vi "PLC_comm.vi"() -> ()   [LabVIEW 2017]
uses:
  <vilib>/DATA AHEAD/SP7/typedefs/PLC Type.ctl
  <vilib>/Utility/error.llb/DialogType.ctl
  <vilib>/addons/database/Connection.llb/DB Tools Open Connec (String).vi
  Global/Global 1.vi
  Global/DATA LOG.vi
  <vilib>/DATA AHEAD/SP7/functions/write/write Dint array.vi
  <vilib>/DATA AHEAD/SP7/functions/write/writeString.vi
  <vilib>/DATA AHEAD/SP7/functions/read/read Dint array.vi
  <vilib>/DATA AHEAD/SP7/functions/read/read real array.vi
  <vilib>/DATA AHEAD/SP7/functions/read/read String.vi
  <vilib>/addons/database/NI_Database_API.lvlib
  <vilib>/DATA AHEAD/SP7/SP7.lvlib
panel:
  out "IP1 7":string
  out "PLC 7":bool
  out "IP1 6":string
  out "PLC 6":bool
  out "IP1 5":string
  out "PLC 5":bool
  out "PLC 4":bool
  out "PLC 3":bool
  out "PLC 2":bool
  out "PLC 1":bool
  out "IP1 4":string
  out "IP1 3":string
  out "IP1 2":string
  out "IP1":string
  in  "stop":bool
  out "error out":errorcluster
  in  "error in (no error)":errorcluster
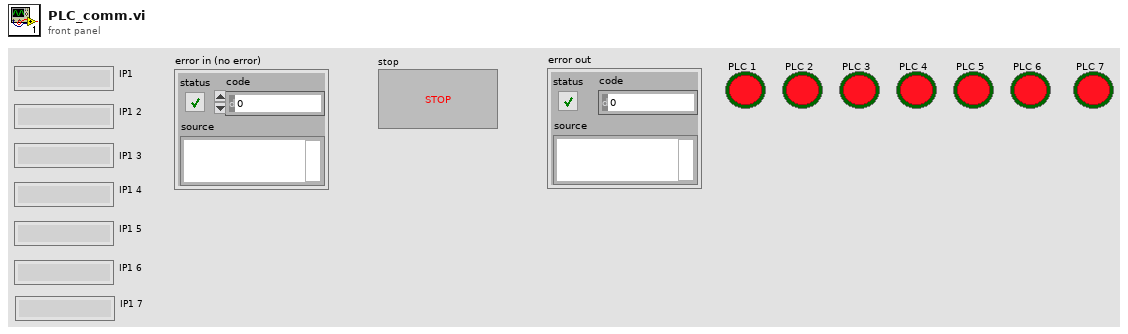
[diagram p1: front panel]
types:
  T1 = typedef "DialogType.ctl" = u16
  T2 = typedef "SP7.lvlib/PLC Type.ctl" = enum16{"S7 200", "S7 300/400", "S7 1200", "S7 1500", "LOGO!8"}
  T3 = typedef "NI_Database_API.lvlib/Conn ObjectReference.ctl" = refnum<k1>
  T4 = typedef "SP7.lvlib/S7 Connection.ctl" = cluster{"TCP Connection Ref":refnum<k5>, "IP address":string, "timeout ms":i32, "Connected?":bool, "PLC Type":T2, "Rack S7 400":u8, "Slot S7 400":u8, "PDU Size":u16, "connection semaphore":T5}
  T5 = typedef "Semaphore RefNum" = refnum<k1>
diagram:
  w2 = T1 0 items=["no dialog", "OK message", "continue or stop message", "OK message + warnings", "continue/stop + warnings"]  # type of dialog (OK msg:1)
  w4 = i32[] [0, 0, 0, 0, 0]  # I/P
  w5 = i32[] [0, 0]  # Input
  w7 = i32[] [0, 0]  # Input
  w8 = i32[] [0, 0]  # Input
  w10 = i32[] [0, 0]  # Input
  w6 = i32[] [0, 0, 0, 0, 0]  # I/P
  w9 = i32[] [0, 0, 0, 0, 0]  # I/P
  w11 = i32[] [0, 0, 0, 0, 0]  # I/P
  w12 = i32[] [0, 0, 0, 0, 0]  # I/P
  w13 = i32[] [0, 0]  # Input
  w14 = i32[] [0, 0]  # Input
  w15 = i32[] [0, 0, 0, 0, 0]  # I/P
  w16 = i32[] [0, 0, 0, 0, 0]  # I/P
  w17 = i32[] [0, 0]  # Input
  w18 = i32[] [0, 0]  # I/P
  w19 = i32[] [0, 0]  # Input
  # "OP 80"
  # "OP 70"
  # "OP 60"
  # "OP 50"
  # "OP 40"
  # "OP 30"
  # "OP 20"
  # "OP 10"
  n1 = call "path_db.vi"("error in"="error in (no error)") -> ("error out"=w174:errorcluster, "resulting string"=w179:string)  [unwired: 9 in]
  n2 = call-poly <vilib>:"DB Tools Open Connection.vi"("error in (no error)"=w174, "connection information"=w179) -> ("error out"=w178:errorcluster, "connection reference"=w177:T3)  [unwired: 6 in]
  n3 = call <vilib>:"DB Tools Select Data.vi"("error in (no error)"=w178, "columns"=string[] ["PLC_IP_1", "PLC_IP_2", "PLC_IP_3", "PLC_IP_4", "PLC_IP_5", "PLC_IP_6", "PLC_IP_7"], "table"="IP_SETTING", "connection reference"=w177) -> ("error out"=w176:errorcluster, "data"=w175:variant[][])  [unwired: 2 in, 1 out]
  n4 = call "PADMINI_varient_to_data.vi"("error in (no error)"=w176, "data"=w175) -> ("error out"=w26:errorcluster, "Array"=w170:string[][])  [unwired: 8 in]
  n5 = call "PADMINI_AUTO_CYCLE STATE.vi"("Enum"=enum16{"Read", "Write"}."Write", "error in (no error)"=w26, "Input"=w19) -> ("error out"=w156:errorcluster)  [unwired: 7 in, 1 out]
  n6 = Index Array(array=w170, index (row)=0) -> (element=w169:string[])  [unwired: 1 in]
  n7 = call "PADMINI_AUTO_BARCODE_STRING.vi"("Enum"=enum16{"Read", "Write"}."Write", "error in (no error)"=w156, "Input"=string[] ["", ""]) -> ("error out"=w153:errorcluster)  [unwired: 7 in, 1 out]
  n8 = call "PADMINI_AUTO_BARCODE_STATUS.vi"("Enum"=enum16{"Read", "Write"}."Write", "error in (no error)"=w153, "I/P"=w18) -> ("error out"=w151:errorcluster)  [unwired: 7 in, 1 out]
  n9 = call "PADMINI_AUTO_CYCLE VALUE 10.vi"("Enum"=enum16{"Read", "Write"}."Write", "error in (no error)"=w151, "Input"=dbl[] [0.0]) -> ("error out"=w145:errorcluster)  [unwired: 7 in, 1 out]
  n10 = call "PADMINI_AUTO_CYCLE STATE 20.vi"("Enum"=enum16{"Read", "Write"}."Write", "error in (no error)"=w145, "Input"=w5) -> ("error out"=w143:errorcluster)  [unwired: 7 in, 1 out]
  n11 = call "PADMINI_AUTO_CYCLE VALUE 20.vi"("Enum"=enum16{"Read", "Write"}."Write", "error in (no error)"=w143, "Input"=dbl[] [0.0, 0.0, 0.0, 0.0]) -> ("error out"=w139:errorcluster)  [unwired: 7 in, 1 out]
  n12 = call "PADMINI_AUTO_BARCODE_STRING2.vi"("Enum"=enum16{"Read", "Write"}."Write", "error in (no error)"=w139, "Input"=string[] ["", "", "", "", "", "", ""]) -> ("error out"=w137:errorcluster)  [unwired: 7 in, 1 out]
  n13 = call "PADMINI_AUTO_BARCODE_STATUS 20.vi"("Enum"=enum16{"Read", "Write"}."Write", "error in (no error)"=w137, "I/P"=w4) -> ("error out"=w131:errorcluster)  [unwired: 7 in, 1 out]
  n14 = call "PADMINI_AUTO_BARCODE_STATUS 30.vi"("Enum"=enum16{"Read", "Write"}."Write", "error in (no error)"=w131, "I/P"=w6) -> ("error out"=w128:errorcluster)  [unwired: 7 in, 1 out]
  n15 = call "PADMINI_AUTO_CYCLE STATE 30.vi"("Enum"=enum16{"Read", "Write"}."Write", "error in (no error)"=w128, "Input"=w7) -> ("error out"=w127:errorcluster)  [unwired: 7 in, 1 out]
  n16 = call "PADMINI_AUTO_CYCLE VALUE 30.vi"("Enum"=enum16{"Read", "Write"}."Write", "error in (no error)"=w127, "Input"=dbl[] [0.0, 0.0]) -> ("error out"=w124:errorcluster)  [unwired: 7 in, 1 out]
  n17 = call "PADMINI_AUTO_BARCODE_STRING 30.vi"("Enum"=enum16{"Read", "Write"}."Write", "error in (no error)"=w124, "Input"=string[] ["", "", ""]) -> ("error out"=w102:errorcluster)  [unwired: 7 in, 1 out]
  n18 = call "PADMINI_AUTO_BARCODE_STATUS 40.vi"("Enum"=enum16{"Read", "Write"}."Write", "error in (no error)"=w102, "I/P"=w9) -> ("error out"=w101:errorcluster)  [unwired: 7 in, 1 out]
  n19 = call "PADMINI_AUTO_CYCLE VALUE 40.vi"("Enum"=enum16{"Read", "Write"}."Write", "error in (no error)"=w101, "Input"=dbl[] [0.0, 0.0, 0.0, 0.0]) -> ("error out"=w100:errorcluster)  [unwired: 7 in, 1 out]
  n20 = call "PADMINI_AUTO_CYCLE STATE 40.vi"("Enum"=enum16{"Read", "Write"}."Write", "error in (no error)"=w100, "Input"=w8) -> ("error out"=w99:errorcluster)  [unwired: 7 in, 1 out]
  n21 = call "PADMINI_AUTO_BARCODE_STRING 40.vi"("Enum"=enum16{"Read", "Write"}."Write", "error in (no error)"=w99, "Input"=string[] ["", "", "", "", ""]) -> ("error out"=w81:errorcluster)  [unwired: 7 in, 1 out]
  n22 = call "PADMINI_AUTO_BARCODE_STATUS 50.vi"("Enum"=enum16{"Read", "Write"}."Write", "error in (no error)"=w81, "I/P"=w11) -> ("error out"=w83:errorcluster)  [unwired: 7 in, 1 out]
  n23 = call "PADMINI_AUTO_CYCLE STATE 50.vi"("Enum"=enum16{"Read", "Write"}."Write", "error in (no error)"=w83, "Input"=w10) -> ("error out"=w87:errorcluster)  [unwired: 7 in, 1 out]
  n24 = call "PADMINI_AUTO_CYCLE VALUE 50.vi"("Enum"=enum16{"Read", "Write"}."Write", "error in (no error)"=w87, "Input"=dbl[] [0.0, 0.0, 0.0]) -> ("error out"=w84:errorcluster)  [unwired: 7 in, 1 out]
  n25 = call "PADMINI_AUTO_BARCODE_STRING 50.vi"("Enum"=enum16{"Read", "Write"}."Write", "error in (no error)"=w84, "Input"=string[] ["", "", "", ""]) -> ("error out"=w59:errorcluster)  [unwired: 7 in, 1 out]
  n26 = call "PADMINI_AUTO_BARCODE_STATUS 60.vi"("Enum"=enum16{"Read", "Write"}."Write", "error in (no error)"=w59, "I/P"=w12) -> ("error out"=w63:errorcluster)  [unwired: 7 in, 1 out]
  n27 = call "PADMINI_AUTO_CYCLE STATE 60.vi"("Enum"=enum16{"Read", "Write"}."Write", "error in (no error)"=w63, "Input"=w13) -> ("error out"=w65:errorcluster)  [unwired: 7 in, 1 out]
  n28 = call "PADMINI_AUTO_CYCLE VALUE 60.vi"("Enum"=enum16{"Read", "Write"}."Write", "error in (no error)"=w65, "Input"=dbl[] [0.0, 0.0, 0.0, 0.0, 0.0]) -> ("error out"=w68:errorcluster)  [unwired: 7 in, 1 out]
  n29 = call "PADMINI_AUTO_BARCODE_STRING 60.vi"("Enum"=enum16{"Read", "Write"}."Write", "error in (no error)"=w68, "Input"=string[] ["", "", "", "", "", ""]) -> ("error out"=w35:errorcluster)  [unwired: 7 in, 1 out]
  n30 = call "PADMINI_AUTO_BARCODE_STATUS 70.vi"("Enum"=enum16{"Read", "Write"}."Write", "error in (no error)"=w35, "I/P"=w15) -> ("error out"=w38:errorcluster)  [unwired: 7 in, 1 out]
  n31 = call "PADMINI_AUTO_CYCLE STATE 70.vi"("Enum"=enum16{"Read", "Write"}."Read", "error in (no error)"=w38, "Input"=w14) -> ("error out"=w50:errorcluster)  [unwired: 7 in, 1 out]
  n32 = call "PADMINI_AUTO_CYCLE VALUE 70.vi"("Enum"=enum16{"Read", "Write"}."Write", "error in (no error)"=w50, "Input"=dbl[] [0.0, 0.0]) -> ("error out"=w47:errorcluster)  [unwired: 7 in, 1 out]
  n33 = call "PADMINI_AUTO_BARCODE_STRING 70.vi"("Enum"=enum16{"Read", "Write"}."Write", "error in (no error)"=w47, "Input"=string[] ["", ""]) -> ("error out"=w32:errorcluster)  [unwired: 7 in, 1 out]
  n34 = call "PADMINI_AUTO_BARCODE_STATUS 80.vi"("Enum"=enum16{"Read", "Write"}."Write", "error in (no error)"=w32, "I/P"=w16) -> ("error out"=w39:errorcluster)  [unwired: 7 in, 1 out]
  n35 = call "PADMINI_AUTO_CYCLE STATE 80.vi"("Enum"=enum16{"Read", "Write"}."Write", "error in (no error)"=w39, "Input"=w17) -> ("error out"=w43:errorcluster)  [unwired: 7 in, 1 out]
  n36 = call "PADMINI_AUTO_CYCLE VALUE 80.vi"("Enum"=enum16{"Read", "Write"}."Write", "error in (no error)"=w43, "Input"=sgl[] [0.0]) -> ("error out"=w46:errorcluster)  [unwired: 7 in, 1 out]
  n37 = call "PADMINI_AUTO_BARCODE_STRING 80.vi"("Enum"=enum16{"Read", "Write"}."Write", "error in (no error)"=w46, "Input"=string[] ["", "", ""]) -> ()  [unwired: 7 in, 2 out]
  n38 = Index Array(array=w169) -> (element #1=w118:string, element #2=w119:string, element #3=w113:string, element #4=w89:string, element #5=w71:string, element #6=w28:string, element #7=w27:string)  [unwired: 7 in]
  "IP1" <- w118
  "IP1 2" <- w119
  "IP1 3" <- w113
  "IP1 4" <- w89
  "IP1 5" <- w71
  "IP1 6" <- w28
  "IP1 7" <- w27
  n39 = call <vilib>:"connect.vi"("PLC Type"=PLC_Type."S7 1200" ("PLC Type 2"), "error in (no error)"=w26, "timeout [ms]"=1000 ("timeout [ms] 2"), "IP address"=w27) -> ("error out"=w29:errorcluster, "S7 Connection out"=w1:T4)  [unwired: 6 in]
  n40 = call <vilib>:"connect.vi"("PLC Type"=PLC_Type."S7 1200" ("PLC Type 2"), "error in (no error)"=w26, "timeout [ms]"=1000 ("timeout [ms] 2"), "IP address"=w71) -> ("error out"=w76:errorcluster, "S7 Connection out"=w75:T4)  [unwired: 6 in]
  n41 = call <vilib>:"connect.vi"("PLC Type"=PLC_Type."S7 1200" ("PLC Type 2"), "error in (no error)"=w26, "timeout [ms]"=1000 ("timeout [ms] 2"), "IP address"=w28) -> ("error out"=w56:errorcluster, "S7 Connection out"=w55:T4)  [unwired: 6 in]
  n42 = call <vilib>:"connect.vi"("PLC Type"=PLC_Type."S7 1200" ("PLC Type 2"), "error in (no error)"=w26, "timeout [ms]"=1000 ("timeout [ms] 2"), "IP address"=w89) -> ("error out"=w92:errorcluster, "S7 Connection out"=w93:T4)  [unwired: 6 in]
  n43 = call <vilib>:"connect.vi"("PLC Type"=PLC_Type."S7 1200" ("PLC Type 2"), "error in (no error)"=w26, "timeout [ms]"=1000 ("timeout [ms] 2"), "IP address"=w119) -> ("error out"=w134:errorcluster, "S7 Connection out"=w133:T4)  [unwired: 6 in]
  n44 = call <vilib>:"connect.vi"("PLC Type"=PLC_Type."S7 1200" ("PLC Type 2"), "error in (no error)"=w26, "timeout [ms]"=1000 ("timeout [ms] 2"), "IP address"=w113) -> ("error out"=w115:errorcluster, "S7 Connection out"=w114:T4)  [unwired: 6 in]
  n45 = call <vilib>:"connect.vi"("PLC Type"=PLC_Type."S7 1200" ("PLC Type 2"), "error in (no error)"=w26, "timeout [ms]"=1000, "IP address"=w118) -> ("error out"=w160:errorcluster, "S7 Connection out"=w159:T4)  [unwired: 6 in]
  n46 = while {
    shift-right: [w182] -> w23
    shift-left: w1 -> [w192]
    shift-right: [w190] -> w24
    shift-left: w29 -> [w191]
    tunnel: w27 -> [w181]
    stop <- w184 stop-if-true
    # "OP 90 - 100 - 110"
    n47 = flat-sequence {
      tunnel: [w267] -> w188
      tunnel: [w268] -> w183
      tunnel: w191 -> [w306]
      tunnel: w192 -> [w305]
      tunnel: w181 -> [w287]
      tunnel: [w287] -> w180
      tunnel: [w374] -> w190
      tunnel: [w373] -> w182
      tunnel: w188 -> [w376]
      tunnel: w183 -> [w375]
      tunnel: w180 -> [w372]
      frame #0 {
        w208 = u16 75 ("Data Block #")
        (unwired) u16 1 ("Items # [byte]")
        w233 = u16 72 ("Data Block #")
        w259 = u16 70 ("Data Block #")
        w217 = u16 71 ("Data Block #")
        w247 = u16 69 ("Data Block #")
        # "OP100 OK\nOP 100 NG"
        # "AUTO WRITE"
        n48 = global read "DATA LOG.vi" "OP 90 Outputs"() -> (w304:bool)
        n49 = case shown="True" w304 {
          tunnel: w305 -> [w357 w370]
          tunnel: [w358 w359] -> w264
          tunnel: [w357 w360] -> w265
          tunnel: w306 -> [w358 w367]
          frame False {
          }
          frame True {
            w371 = u16 70  # Data Block #
            n50 = call "PADMINI_AUTO_BARCODE_STATUS 90.vi"("Enum"=enum16{"Read", "Write"}."Read", "error in (no error)"=w367) -> ("error out"=w366:errorcluster, "O/P"=w368:i32[])  [unwired: 8 in]
            n51 = global write "DATA LOG.vi" "OP 90 Outputs"(FALSE) -> ()
            n52 = call-poly <vilib>:"write DB.vi"("DINT input array"=w368, "error in (no error)"=w366, "Data Block #"=w371, "S7 Connection in"=w370) -> ("error out"=w362:errorcluster, "S7 Connection out"=w361:T4)  [unwired: 4 in, 2 out]
            n53 = call-poly <vilib>:"write DB.vi"("DINT input array"=i32[] [0] ("Data Byte"), "error in (no error)"=w362, "Data Block #"=u16 69, "S7 Connection in"=w361) -> ("error out"=w359:errorcluster, "S7 Connection out"=w360:T4)  [unwired: 4 in, 2 out]
          }
        }
        n54 = global read "DATA LOG.vi" "OP 90 reset"() -> (w263:bool)
        n55 = case shown="True" w263 {
          tunnel: w264 -> [w332 w341]
          tunnel: [w332 w340] -> w252
          tunnel: w265 -> [w333 w339]
          tunnel: [w333 w338] -> w253
          frame False {
          }
          frame True {
            n56 = global write "DATA LOG.vi" "OP 90 reset"(FALSE) -> ()
            n57 = call-poly <vilib>:"write DB.vi"("Item offset [byte]"=u16 4 ("Data Block #"), "DINT input array"=i32[] [0], "error in (no error)"=w341, "Data Block #"=u16 69, "S7 Connection in"=w339) -> ("error out"=w340:errorcluster, "S7 Connection out"=w338:T4)  [unwired: 3 in, 2 out]
          }
        }
        n58 = global read "DATA LOG.vi" "Auto Cycle On"() -> (w199:bool)
        n59 = Boolean To (0,1)(Boolean=w199) -> (0, 1=w198:i16)
        n60 = Build Array(w198) -> (w197:i16[])
        n61 = global read "Global 1.vi" "Filtered BARCODE selected"() -> (w262:string[])
        n62 = call-poly <vilib>:"write DB.vi"("Item offset [byte]"=u32 20, "DINT input array"=w197, "error in (no error)"=w252, "Data Block #"=w259, "S7 Connection in"=w253) -> ("error out"=w257:errorcluster, "S7 Connection out"=w256:T4)  [unwired: 3 in, 2 out]
        n63 = call-poly <vilib>:"write DB.vi"("Item offset [byte]"=u32 24, "Input STRINGS"=w262, "error in (no error)"=w257, "String length reserved in DB (default=254)"=u16 15, "Data Block #"=w259, "S7 Connection in"=w256) -> ("error out"=w254:errorcluster, "S7 Connection out"=w255:T4)  [unwired: 2 in, 2 out]
        n64 = call-poly <vilib>:"read DB.vi"("error in (no error)"=w254, "items #"=u16 2 ("Items # [byte]"), "Data Block #"=w247, "S7 Connection in"=w255) -> ("error out"=w302:errorcluster, "DINT result array"=w300:i32[], "S7 Connection out"=w297:T4)  [unwired: 5 in]
        n65 = call "PADMINI_AUTO_CYCLE STATE 90.vi"("Enum"=enum16{"Read", "Write"}."Write", "error in (no error)"=w302, "Input"=w300) -> ("error out"=w298:errorcluster)  [unwired: 7 in, 1 out]
        n66 = call-poly <vilib>:"read DB.vi"("Item offset [byte]"=u32 8, "error in (no error)"=w298, "items #"=u16 2 ("Items # [byte]"), "Data Block #"=w247, "S7 Connection in"=w297) -> ("error out"=w290:errorcluster, "REAL result array"=w288:sgl[], "S7 Connection out"=w296:T4)  [unwired: 4 in]
        n67 = call "PADMINI_AUTO_CYCLE VALUE 90.vi"("Enum"=enum16{"Read", "Write"}."Write", "error in (no error)"=w290, "Input"=w288) -> ("error out"=w289:errorcluster)  [unwired: 7 in, 1 out]
        n68 = call-poly <vilib>:"read DB.vi"("Item offset [byte]"=u32 16, "String length reserved in DB (default=254)"=u16 50, "error in (no error)"=w289, "items #"=u16 1 ("Items # [byte]"), "Data Block #"=w247, "S7 Connection in"=w296) -> ("error out"=w251:errorcluster, "STRING result Array"=w242:string[], "S7 Connection out"=w250:T4)  [unwired: 2 in, 1 out]
        n69 = call-poly <vilib>:"read DB.vi"("Item offset [byte]"=u32 68, "String length reserved in DB (default=254)"=u16 10, "error in (no error)"=w251, "items #"=u16 3 ("Items # [byte]"), "Data Block #"=w247, "S7 Connection in"=w250) -> ("error out"=w249:errorcluster, "STRING result Array"=w241:string[], "S7 Connection out"=w248:T4)  [unwired: 2 in, 1 out]
        n70 = Build Array (concatenate)(w242, w241) -> (w240:string[])
        n71 = call "PADMINI_AUTO_BARCODE_STRING 90.vi"("Enum"=enum16{"Read", "Write"}."Write", "error in (no error)"=w249, "Input"=w240) -> ("error out"=w269:errorcluster)  [unwired: 7 in, 1 out]
        n72 = global read "DATA LOG.vi" "OP 100 Outputs"() -> (w270:bool)
        n73 = case shown="True" w270 {
          tunnel: w248 -> [w342 w355]
          tunnel: [w343 w346] -> w238
          tunnel: [w342 w347] -> w239
          tunnel: w269 -> [w343 w352]
          frame False {
          }
          frame True {
            w356 = u16 72  # Data Block #
            n74 = call "PADMINI_AUTO_BARCODE_STATUS 100.vi"("Enum"=enum16{"Read", "Write"}."Read", "error in (no error)"=w352) -> ("error out"=w351:errorcluster, "O/P"=w353:i32[])  [unwired: 8 in]
            n75 = global write "DATA LOG.vi" "OP 100 Outputs"(FALSE) -> ()
            n76 = call-poly <vilib>:"write DB.vi"("DINT input array"=w353, "error in (no error)"=w351, "Data Block #"=w356, "S7 Connection in"=w355) -> ("error out"=w345:errorcluster, "S7 Connection out"=w344:T4)  [unwired: 4 in, 2 out]
            n77 = call-poly <vilib>:"write DB.vi"("DINT input array"=i32[] [0] ("Data Byte"), "error in (no error)"=w345, "Data Block #"=u16 71, "S7 Connection in"=w344) -> ("error out"=w346:errorcluster, "S7 Connection out"=w347:T4)  [unwired: 4 in, 2 out]
          }
        }
        n78 = global read "DATA LOG.vi" "OP 100 reset"() -> (w237:bool)
        n79 = case shown="True" w237 {
          tunnel: w238 -> [w322 w331]
          tunnel: [w322 w330] -> w229
          tunnel: w239 -> [w323 w329]
          tunnel: [w323 w328] -> w228
          frame False {
          }
          frame True {
            n80 = global write "DATA LOG.vi" "OP 100 reset"(FALSE) -> ()
            n81 = call-poly <vilib>:"write DB.vi"("Item offset [byte]"=u16 4 ("Data Block #"), "DINT input array"=i32[] [0], "error in (no error)"=w331, "Data Block #"=u16 71, "S7 Connection in"=w329) -> ("error out"=w330:errorcluster, "S7 Connection out"=w328:T4)  [unwired: 3 in, 2 out]
          }
        }
        n82 = global read "DATA LOG.vi" "Auto Cycle On"() -> (w196:bool)
        n83 = Boolean To (0,1)(Boolean=w196) -> (0, 1=w195:i16)
        n84 = Build Array(w195) -> (w194:i16[])
        n85 = global read "Global 1.vi" "Filtered BARCODE selected"() -> (w230:string[])
        n86 = call-poly <vilib>:"write DB.vi"("Item offset [byte]"=u32 20, "DINT input array"=w194, "error in (no error)"=w229, "Data Block #"=w233, "S7 Connection in"=w228) -> ("error out"=w235:errorcluster, "S7 Connection out"=w236:T4)  [unwired: 3 in, 2 out]
        n87 = call-poly <vilib>:"write DB.vi"("Item offset [byte]"=u32 24, "Input STRINGS"=w230, "error in (no error)"=w235, "String length reserved in DB (default=254)"=u16 15, "Data Block #"=w233, "S7 Connection in"=w236) -> ("error out"=w226:errorcluster, "S7 Connection out"=w227:T4)  [unwired: 2 in, 2 out]
        n88 = call-poly <vilib>:"read DB.vi"("error in (no error)"=w226, "items #"=u16 2 ("Items # [byte]"), "Data Block #"=w217, "S7 Connection in"=w227) -> ("error out"=w272:errorcluster, "DINT result array"=w274:i32[], "S7 Connection out"=w277:T4)  [unwired: 5 in]
        n89 = call "PADMINI_AUTO_CYCLE STATE 100.vi"("Enum"=enum16{"Read", "Write"}."Write", "error in (no error)"=w272, "Input"=w274) -> ("error out"=w276:errorcluster)  [unwired: 7 in, 1 out]
        n90 = call-poly <vilib>:"read DB.vi"("Item offset [byte]"=u32 8, "error in (no error)"=w276, "items #"=u16 11 ("Items # [byte]"), "Data Block #"=w217, "S7 Connection in"=w277) -> ("error out"=w284:errorcluster, "REAL result array"=w286:sgl[], "S7 Connection out"=w278:T4)  [unwired: 4 in]
        n91 = call "PADMINI_AUTO_CYCLE VALUE 100.vi"("Enum"=enum16{"Read", "Write"}."Write", "error in (no error)"=w284, "Input"=w286) -> ("error out"=w285:errorcluster)  [unwired: 7 in, 1 out]
        n92 = call-poly <vilib>:"read DB.vi"("Item offset [byte]"=u32 52, "String length reserved in DB (default=254)"=u16 50, "error in (no error)"=w285, "items #"=u16 1 ("Items # [byte]"), "Data Block #"=w217, "S7 Connection in"=w278) -> ("error out"=w223:errorcluster, "STRING result Array"=w220:string[], "S7 Connection out"=w222:T4)  [unwired: 2 in, 1 out]
        n93 = call-poly <vilib>:"read DB.vi"("Item offset [byte]"=u32 104, "String length reserved in DB (default=254)"=u16 10, "error in (no error)"=w223, "Data Block #"=w217, "S7 Connection in"=w222) -> ("error out"=w224:errorcluster, "STRING result Array"=w218:string[], "S7 Connection out"=w221:T4)  [unwired: 3 in, 1 out]
        n94 = Build Array (concatenate)(w220, w218) -> (w219:string[])
        n95 = call "PADMINI_AUTO_BARCODE_STRING 100.vi"("Enum"=enum16{"Read", "Write"}."Write", "error in (no error)"=w224, "Input"=w219) -> ("error out"=w266:errorcluster)  [unwired: 7 in, 1 out]
        n96 = global read "DATA LOG.vi" "OP 110 Outputs"() -> (w214:bool)
        n97 = case shown="True" w214 {
          tunnel: [w307 w312] -> w200
          tunnel: [w308 w313] -> w201
          tunnel: w266 -> [w307 w317]
          tunnel: w221 -> [w308 w316]
          frame False {
          }
          frame True {
            w309 = i32[] [0]  # DINT input array
            w310 = u16 75  # Data Block #
            n98 = call "PADMINI_AUTO_BARCODE_STATUS 110.vi"("Enum"=enum16{"Read", "Write"}."Read", "error in (no error)"=w317) -> ("error out"=w319:errorcluster, "O/P"=w320:i32[])  [unwired: 8 in]
            n99 = call-poly <vilib>:"write DB.vi"("Item offset [byte]"=u32 4, "DINT input array"=w320, "error in (no error)"=w319, "Data Block #"=w310, "S7 Connection in"=w316) -> ("error out"=w311:errorcluster, "S7 Connection out"=w314:T4)  [unwired: 3 in, 2 out]
            n100 = global write "DATA LOG.vi" "OP 110 Outputs"(FALSE) -> ()
            n101 = call-poly <vilib>:"write DB.vi"("DINT input array"=w309, "error in (no error)"=w311, "Data Block #"=w310, "S7 Connection in"=w314) -> ("error out"=w312:errorcluster, "S7 Connection out"=w313:T4)  [unwired: 4 in, 2 out]
          }
        }
        n102 = call-poly <vilib>:"read DB.vi"("error in (no error)"=w200, "items #"=u16 1 ("Items # [byte]"), "Data Block #"=w208, "S7 Connection in"=w201) -> ("error out"=w212:errorcluster, "DINT result array"=w210:i32[], "S7 Connection out"=w209:T4)  [unwired: 5 in]
        n103 = call "PADMINI_AUTO_CYCLE STATE 110.vi"("Enum"=enum16{"Read", "Write"}."Write", "error in (no error)"=w212, "Input"=w210) -> ("error out"=w202:errorcluster)  [unwired: 7 in, 1 out]
        n104 = call-poly <vilib>:"read DB.vi"("Item offset [byte]"=u32 12, "String length reserved in DB (default=254)"=u16 50, "error in (no error)"=w202, "items #"=u16 1 ("Items # [byte]"), "Data Block #"=w208, "S7 Connection in"=w209) -> ("error out"=w204:errorcluster, "STRING result Array"=w205:string[], "S7 Connection out"=w267:T4)  [unwired: 2 in, 1 out]
        n105 = call "PADMINI_AUTO_BARCODE_STRING 110.vi"("Enum"=enum16{"Read", "Write"}."Write", "error in (no error)"=w204, "Input"=w205) -> ("error out"=w268:errorcluster)  [unwired: 7 in, 1 out]
      }
      frame #1 {
        # "RECONNECT"
        n106 = case shown="Error" w375 {
          selector: w375 -> [w380 w388]
          tunnel: [w379 w385] -> w373
          tunnel: [w380 w386] -> w374
          tunnel: w376 -> [w379 w382]
          tunnel: w372 -> [_ w381]
          frame No Error {
          }
          frame Error {
            n107 = call <vilib>:"Clear Errors.vi"("error in (no error)"=w388) -> ("error out"=w389:errorcluster)  [unwired: 5 in, 1 out]
            n108 = call <vilib>:"disconnect.vi"("error in (no error)"=w389, "S7 Connection in"=w382) -> ("error out"=w387:errorcluster)  [unwired: 8 in, 1 out]
            n109 = call <vilib>:"Clear Errors.vi"("error in (no error)"=w387) -> ("error out"=w384:errorcluster)  [unwired: 5 in, 1 out]
            n110 = call <vilib>:"connect.vi"("PLC Type"=PLC_Type."S7 1200" ("PLC Type 2"), "error in (no error)"=w384, "IP address"=w381) -> ("error out"=w386:errorcluster, "S7 Connection out"=w385:T4)  [unwired: 7 in]
          }
        }
        n111 = Unbundle By Name(w375) -> ("status"=w378:bool)
        n112 = Not(x=w378) -> (.not. x?=w377:bool)
        "PLC 7" <- w377
        n113 = global write "Global 1.vi" "PLC 7"(w377) -> ()
      }
    }
    n114 = call "PADMINI_STOP_ALL.vi"("Enum"=enum16{"Read", "Write"}."Read") -> ("Boolean 2"=w186:bool)  [unwired: 9 in, 1 out]
    n115 = local read "stop"() -> (w185:bool)
    n116 = Or(x=w185, y=w186) -> (x .or. y?=w184:bool)
    n117 = Wait (ms)(milliseconds to wait=u32 50) -> ()  [unwired: 1 out]
  }
  n118 = while {
    shift-right: [w392] -> w121
    shift-left: w133 -> [w402]
    shift-right: [w400] -> w120
    shift-left: w134 -> [w401]
    tunnel: w119 -> [w391]
    stop <- w394 stop-if-true
    # "OP 30"
    n119 = flat-sequence {
      tunnel: [w405] -> w398
      tunnel: [w407] -> w393
      tunnel: w401 -> [w409]
      tunnel: w402 -> [w408]
      tunnel: w391 -> [w406]
      tunnel: [w406] -> w390
      tunnel: [w412] -> w400
      tunnel: [w411] -> w392
      tunnel: w398 -> [w414]
      tunnel: w393 -> [w413]
      tunnel: w390 -> [w410]
      frame #0 {
        # "AUTO WRITE"
        n120 = call "PLC_OP30_Write.vi"("error in (no error)"=w409, "S7 Connection in"=w408) -> ("error out"=w403:errorcluster, "S7 Connection out"=w404:T4)  [unwired: 8 in]
        n121 = call "PLC_OP30_Read.vi"("error in (no error)"=w403, "S7 Connection in"=w404) -> ("error out"=w407:errorcluster, "S7 Connection out 2"=w405:T4)  [unwired: 8 in]
      }
      frame #1 {
        # "RECONNECT"
        n122 = case shown="Error" w413 {
          selector: w413 -> [w418 w426]
          tunnel: [w417 w423] -> w411
          tunnel: [w418 w424] -> w412
          tunnel: w414 -> [w417 w420]
          tunnel: w410 -> [_ w419]
          frame No Error {
          }
          frame Error {
            n123 = call <vilib>:"Clear Errors.vi"("error in (no error)"=w426) -> ("error out"=w427:errorcluster)  [unwired: 5 in, 1 out]
            n124 = call <vilib>:"disconnect.vi"("error in (no error)"=w427, "S7 Connection in"=w420) -> ("error out"=w425:errorcluster)  [unwired: 8 in, 1 out]
            n125 = call <vilib>:"Clear Errors.vi"("error in (no error)"=w425) -> ("error out"=w422:errorcluster)  [unwired: 5 in, 1 out]
            n126 = call <vilib>:"connect.vi"("PLC Type"=PLC_Type."S7 1200" ("PLC Type 2"), "error in (no error)"=w422, "IP address"=w419) -> ("error out"=w424:errorcluster, "S7 Connection out"=w423:T4)  [unwired: 7 in]
          }
        }
        n127 = Unbundle By Name(w413) -> ("status"=w416:bool)
        n128 = Not(x=w416) -> (.not. x?=w415:bool)
        "PLC 2" <- w415
        n129 = global write "Global 1.vi" "PLC 2"(w415) -> ()
      }
    }
    n130 = call "PADMINI_STOP_ALL.vi"("Enum"=enum16{"Read", "Write"}."Read") -> ("Boolean 2"=w396:bool)  [unwired: 9 in, 1 out]
    n131 = Wait (ms)(milliseconds to wait=u32 50) -> ()  [unwired: 1 out]
    n132 = local read "stop"() -> (w395:bool)
    n133 = Or(x=w395, y=w396) -> (x .or. y?=w394:bool)
  }
  n134 = while {
    shift-right: [w430] -> w148
    shift-left: w159 -> [w440]
    shift-right: [w438] -> w163
    shift-left: w160 -> [w439]
    tunnel: w118 -> [w428]
    stop <- w433 stop-if-true
    # "OP 10 AND 20"
    n135 = flat-sequence {
      tunnel: [w443] -> w432
      tunnel: [w449] -> w431
      tunnel: w439 -> [w450]
      tunnel: w440 -> [w451]
      tunnel: [w448] -> w429
      tunnel: w428 -> [w448]
      tunnel: [w455] -> w438
      tunnel: [w454] -> w430
      tunnel: w432 -> [w456]
      tunnel: w431 -> [w452]
      tunnel: w429 -> [w453]
      frame #0 {
        # "NEW CHANGES"
        n136 = call "PLC_OP10_Write.vi"("error in (no error)"=w450, "S7 Connection in"=w451) -> ("error out"=w446:errorcluster, "S7 Connection out"=w447:T4)  [unwired: 8 in]
        n137 = call "PLC_OP10_Read.vi"("error in (no error)"=w446, "S7 Connection in"=w447) -> ("error out"=w445:errorcluster, "S7 Connection out"=w444:T4)  [unwired: 8 in]
        n138 = call "PLC_OP20_Write.vi"("error in (no error)"=w445, "S7 Connection in"=w444) -> ("error out"=w441:errorcluster, "S7 Connection out"=w442:T4)  [unwired: 8 in]
        n139 = call "PLC_OP20_Read.vi"("error in (no error)"=w441, "S7 Connection in"=w442) -> ("error out"=w449:errorcluster, "S7 Connection out 2"=w443:T4)  [unwired: 8 in]
      }
      frame #1 {
        # "RECONNECT"
        n140 = Unbundle By Name(w452) -> ("status"=w458:bool)
        n141 = case shown="Error" w452 {
          selector: w452 -> [w460 w469]
          tunnel: [w459 w466] -> w454
          tunnel: [w460 w467] -> w455
          tunnel: w456 -> [w459 w463]
          tunnel: w453 -> [_ w462]
          frame No Error {
          }
          frame Error {
            w461 = 1000  # timeout [ms]
            n142 = call <vilib>:"Clear Errors.vi"("error in (no error)"=w469) -> ("error out"=w470:errorcluster)  [unwired: 5 in, 1 out]
            n143 = call <vilib>:"disconnect.vi"("error in (no error)"=w470, "S7 Connection in"=w463) -> ("error out"=w468:errorcluster)  [unwired: 8 in, 1 out]
            n144 = call <vilib>:"Clear Errors.vi"("error in (no error)"=w468) -> ("error out"=w465:errorcluster)  [unwired: 5 in, 1 out]
            n145 = call <vilib>:"connect.vi"("PLC Type"=PLC_Type."S7 1200" ("PLC Type 2"), "error in (no error)"=w465, "timeout [ms]"=w461, "IP address"=w462) -> ("error out"=w467:errorcluster, "S7 Connection out"=w466:T4)  [unwired: 6 in]
          }
        }
        n146 = Not(x=w458) -> (.not. x?=w457:bool)
        "PLC 1" <- w457
        n147 = global write "Global 1.vi" "PLC 1"(w457) -> ()
      }
    }
    n148 = call "PADMINI_STOP_ALL.vi"("Enum"=enum16{"Read", "Write"}."Read") -> ("Boolean 2"=w435:bool)  [unwired: 9 in, 1 out]
    n149 = Or(x="stop", y=w435) -> (x .or. y?=w433:bool)
    n150 = Wait (ms)(milliseconds to wait=u32 50) -> ()  [unwired: 1 out]
  }
  n151 = while {
    shift-right: [w473] -> w96
    shift-left: w93 -> [w483]
    shift-right: [w481] -> w95
    shift-left: w92 -> [w482]
    tunnel: w89 -> [w472]
    stop <- w475 stop-if-true
    # "OP 50"
    n152 = flat-sequence {
      tunnel: [w504] -> w479
      tunnel: [w514] -> w474
      tunnel: w482 -> [w533]
      tunnel: w483 -> [w532]
      tunnel: w472 -> [w513]
      tunnel: [w513] -> w471
      tunnel: [w561] -> w481
      tunnel: [w560] -> w473
      tunnel: w479 -> [w563]
      tunnel: w474 -> [w562]
      tunnel: w471 -> [w559]
      frame #0 {
        w495 = u16 57 ("Data Block #")
        w503 = u16 56 ("Data Block #")
        # "AUTO WRITE"
        n153 = global read "DATA LOG.vi" "OP 50 Outputs"() -> (w531:bool)
        n154 = case shown="True" w531 {
          tunnel: w532 -> [w544 w557]
          tunnel: [w545 w546] -> w512
          tunnel: [w544 w549] -> w511
          tunnel: w533 -> [w545 w554]
          frame False {
          }
          frame True {
            w558 = u16 57  # Data Block #
            n155 = call "PADMINI_AUTO_BARCODE_STATUS 50.vi"("Enum"=enum16{"Read", "Write"}."Read", "error in (no error)"=w554) -> ("error out"=w553:errorcluster, "O/P"=w555:i32[])  [unwired: 8 in]
            n156 = global write "DATA LOG.vi" "OP 50 Outputs"(FALSE) -> ()
            n157 = call-poly <vilib>:"write DB.vi"("DINT input array"=w555, "error in (no error)"=w553, "Data Block #"=w558, "S7 Connection in"=w557) -> ("error out"=w547:errorcluster, "S7 Connection out"=w548:T4)  [unwired: 4 in, 2 out]
            n158 = call-poly <vilib>:"write DB.vi"("DINT input array"=i32[] [0] ("Data Byte"), "error in (no error)"=w547, "Data Block #"=u16 56, "S7 Connection in"=w548) -> ("error out"=w546:errorcluster, "S7 Connection out"=w549:T4)  [unwired: 4 in, 2 out]
          }
        }
        n159 = global read "DATA LOG.vi" "OP 50 reset"() -> (w510:bool)
        n160 = global read "DATA LOG.vi" "Auto Cycle On"() -> (w486:bool)
        n161 = case shown="True" w510 {
          tunnel: w512 -> [w534 w543]
          tunnel: [w534 w542] -> w488
          tunnel: w511 -> [w535 w541]
          tunnel: [w535 w540] -> w491
          frame False {
          }
          frame True {
            n162 = global write "DATA LOG.vi" "OP 50 reset"(FALSE) -> ()
            n163 = call-poly <vilib>:"write DB.vi"("Item offset [byte]"=u16 4 ("Data Block #"), "DINT input array"=i32[] [0], "error in (no error)"=w543, "Data Block #"=u16 56, "S7 Connection in"=w541) -> ("error out"=w542:errorcluster, "S7 Connection out"=w540:T4)  [unwired: 3 in, 2 out]
          }
        }
        n164 = Boolean To (0,1)(Boolean=w486) -> (0, 1=w485:i16)
        n165 = Build Array(w485) -> (w484:i16[])
        n166 = global read "Global 1.vi" "Filtered BARCODE selected"() -> (w492:string[])
        n167 = call-poly <vilib>:"write DB.vi"("Item offset [byte]"=u32 20, "DINT input array"=w484, "error in (no error)"=w488, "Data Block #"=w495, "S7 Connection in"=w491) -> ("error out"=w497:errorcluster, "S7 Connection out"=w498:T4)  [unwired: 3 in, 2 out]
        n168 = call-poly <vilib>:"write DB.vi"("Item offset [byte]"=u32 24, "Input STRINGS"=w492, "error in (no error)"=w497, "String length reserved in DB (default=254)"=u16 15, "Data Block #"=w495, "S7 Connection in"=w498) -> ("error out"=w489:errorcluster, "S7 Connection out"=w490:T4)  [unwired: 2 in, 2 out]
        n169 = call-poly <vilib>:"read DB.vi"("error in (no error)"=w489, "items #"=u16 2 ("Items # [byte]"), "Data Block #"=w503, "S7 Connection in"=w490) -> ("error out"=w529:errorcluster, "DINT result array"=w527:i32[], "S7 Connection out"=w524:T4)  [unwired: 5 in]
        n170 = call "PADMINI_AUTO_CYCLE STATE 50.vi"("Enum"=enum16{"Read", "Write"}."Write", "error in (no error)"=w529, "Input"=w527) -> ("error out"=w525:errorcluster)  [unwired: 7 in, 1 out]
        n171 = call-poly <vilib>:"read DB.vi"("Item offset [byte]"=u32 8, "error in (no error)"=w525, "items #"=u16 3 ("Items # [byte]"), "Data Block #"=w503, "S7 Connection in"=w524) -> ("error out"=w517:errorcluster, "REAL result array"=w515:sgl[], "S7 Connection out"=w523:T4)  [unwired: 4 in]
        n172 = call "PADMINI_AUTO_CYCLE VALUE 50.vi"("Enum"=enum16{"Read", "Write"}."Write", "error in (no error)"=w517, "Input"=w515) -> ("error out"=w516:errorcluster)  [unwired: 7 in, 1 out]
        n173 = call-poly <vilib>:"read DB.vi"("Item offset [byte]"=u32 20, "String length reserved in DB (default=254)"=u16 50, "error in (no error)"=w516, "items #"=u16 1 ("Items # [byte]"), "Data Block #"=w503, "S7 Connection in"=w523) -> ("error out"=w506:errorcluster, "STRING result Array"=w502:string[], "S7 Connection out"=w505:T4)  [unwired: 2 in, 1 out]
        n174 = call-poly <vilib>:"read DB.vi"("Item offset [byte]"=u32 72, "String length reserved in DB (default=254)"=u16 10, "error in (no error)"=w506, "items #"=u16 5 ("Items # [byte]"), "Data Block #"=w503, "S7 Connection in"=w505) -> ("error out"=w507:errorcluster, "STRING result Array"=w501:string[], "S7 Connection out"=w504:T4)  [unwired: 2 in, 1 out]
        n175 = Build Array (concatenate)(w502, w501) -> (w500:string[])
        n176 = call "PADMINI_AUTO_BARCODE_STRING 50.vi"("Enum"=enum16{"Read", "Write"}."Write", "error in (no error)"=w507, "Input"=w500) -> ("error out"=w514:errorcluster)  [unwired: 7 in, 1 out]
      }
      frame #1 {
        # "RECONNECT"
        n177 = case shown="Error" w562 {
          selector: w562 -> [w567 w575]
          tunnel: [w566 w572] -> w560
          tunnel: [w567 w573] -> w561
          tunnel: w563 -> [w566 w569]
          tunnel: w559 -> [_ w568]
          frame No Error {
          }
          frame Error {
            n178 = call <vilib>:"Clear Errors.vi"("error in (no error)"=w575) -> ("error out"=w576:errorcluster)  [unwired: 5 in, 1 out]
            n179 = call <vilib>:"disconnect.vi"("error in (no error)"=w576, "S7 Connection in"=w569) -> ("error out"=w574:errorcluster)  [unwired: 8 in, 1 out]
            n180 = call <vilib>:"Clear Errors.vi"("error in (no error)"=w574) -> ("error out"=w571:errorcluster)  [unwired: 5 in, 1 out]
            n181 = call <vilib>:"connect.vi"("PLC Type"=PLC_Type."S7 1200" ("PLC Type 2"), "error in (no error)"=w571, "IP address"=w568) -> ("error out"=w573:errorcluster, "S7 Connection out"=w572:T4)  [unwired: 7 in]
          }
        }
        n182 = Unbundle By Name(w562) -> ("status"=w565:bool)
        n183 = Not(x=w565) -> (.not. x?=w564:bool)
        "PLC 4" <- w564
        n184 = global write "Global 1.vi" "PLC 4"(w564) -> ()
      }
    }
    n185 = call "PADMINI_STOP_ALL.vi"("Enum"=enum16{"Read", "Write"}."Read") -> ("Boolean 2"=w477:bool)  [unwired: 9 in, 1 out]
    n186 = local read "stop"() -> (w476:bool)
    n187 = Or(x=w476, y=w477) -> (x .or. y?=w475:bool)
    n188 = Wait (ms)(milliseconds to wait=u32 50) -> ()  [unwired: 1 out]
  }
  n189 = while {
    shift-right: [w579] -> w52
    shift-left: w55 -> [w589]
    shift-right: [w587] -> w53
    shift-left: w56 -> [w588]
    tunnel: w28 -> [w578]
    stop <- w581 stop-if-true
    # "OP 70 - 80"
    n190 = flat-sequence {
      tunnel: [w600] -> w585
      tunnel: [w648] -> w580
      tunnel: w588 -> [w686]
      tunnel: w589 -> [w685]
      tunnel: w578 -> [w667]
      tunnel: [w667] -> w577
      tunnel: [w739] -> w587
      tunnel: [w738] -> w579
      tunnel: w585 -> [w741]
      tunnel: w580 -> [w740]
      tunnel: w577 -> [w737]
      frame #0 {
        w616 = u16 83 ("Data Block #")
        w641 = u16 81 ("Data Block #")
        w599 = u16 82 ("Data Block #")
        w622 = u16 80 ("Data Block #")
        # "AUTO WRITE"
        n191 = global read "DATA LOG.vi" "OP 70 Outputs"() -> (w684:bool)
        n192 = case shown="True" w684 {
          tunnel: w685 -> [w722 w735]
          tunnel: [w723 w726] -> w646
          tunnel: [w722 w727] -> w645
          tunnel: w686 -> [w723 w732]
          frame False {
          }
          frame True {
            w736 = u16 81  # Data Block #
            n193 = call "PADMINI_AUTO_BARCODE_STATUS 70.vi"("Enum"=enum16{"Read", "Write"}."Read", "error in (no error)"=w732) -> ("error out"=w731:errorcluster, "O/P"=w733:i32[])  [unwired: 8 in]
            n194 = global write "DATA LOG.vi" "OP 70 Outputs"(FALSE) -> ()
            n195 = call-poly <vilib>:"write DB.vi"("DINT input array"=w733, "error in (no error)"=w731, "Data Block #"=w736, "S7 Connection in"=w735) -> ("error out"=w724:errorcluster, "S7 Connection out"=w725:T4)  [unwired: 4 in, 2 out]
            n196 = call-poly <vilib>:"write DB.vi"("DINT input array"=i32[] [0] ("Data Byte"), "error in (no error)"=w724, "Data Block #"=u16 80, "S7 Connection in"=w725) -> ("error out"=w726:errorcluster, "S7 Connection out"=w727:T4)  [unwired: 4 in, 2 out]
          }
        }
        n197 = global read "DATA LOG.vi" "OP 70 reset"() -> (w647:bool)
        n198 = global read "DATA LOG.vi" "Auto Cycle On"() -> (w592:bool)
        n199 = case shown="True" w647 {
          tunnel: w646 -> [w697 w706]
          tunnel: [w697 w705] -> w636
          tunnel: w645 -> [w698 w704]
          tunnel: [w698 w703] -> w637
          frame False {
          }
          frame True {
            n200 = global write "DATA LOG.vi" "OP 70 reset"(FALSE) -> ()
            n201 = call-poly <vilib>:"write DB.vi"("Item offset [byte]"=u16 4 ("Data Block #"), "DINT input array"=i32[] [0], "error in (no error)"=w706, "Data Block #"=u16 80, "S7 Connection in"=w704) -> ("error out"=w705:errorcluster, "S7 Connection out"=w703:T4)  [unwired: 3 in, 2 out]
          }
        }
        n202 = Boolean To (0,1)(Boolean=w592) -> (0, 1=w591:i16)
        n203 = Build Array(w591) -> (w590:i16[])
        n204 = global read "Global 1.vi" "Filtered BARCODE selected"() -> (w638:string[])
        n205 = call-poly <vilib>:"write DB.vi"("Item offset [byte]"=u32 20, "DINT input array"=w590, "error in (no error)"=w636, "Data Block #"=w641, "S7 Connection in"=w637) -> ("error out"=w643:errorcluster, "S7 Connection out"=w644:T4)  [unwired: 3 in, 2 out]
        n206 = call-poly <vilib>:"write DB.vi"("Item offset [byte]"=u32 24, "Input STRINGS"=w638, "error in (no error)"=w643, "String length reserved in DB (default=254)"=u16 15, "Data Block #"=w641, "S7 Connection in"=w644) -> ("error out"=w634:errorcluster, "S7 Connection out"=w635:T4)  [unwired: 2 in, 2 out]
        n207 = call-poly <vilib>:"read DB.vi"("error in (no error)"=w634, "items #"=u16 2 ("Items # [byte]"), "Data Block #"=w622, "S7 Connection in"=w635) -> ("error out"=w682:errorcluster, "DINT result array"=w680:i32[], "S7 Connection out"=w677:T4)  [unwired: 5 in]
        n208 = call "PADMINI_AUTO_CYCLE STATE 70.vi"("Enum"=enum16{"Read", "Write"}."Write", "error in (no error)"=w682, "Input"=w680) -> ("error out"=w678:errorcluster)  [unwired: 7 in, 1 out]
        n209 = call-poly <vilib>:"read DB.vi"("Item offset [byte]"=u32 8, "error in (no error)"=w678, "items #"=u16 2 ("Items # [byte]"), "Data Block #"=w622, "S7 Connection in"=w677) -> ("error out"=w670:errorcluster, "REAL result array"=w668:sgl[], "S7 Connection out"=w676:T4)  [unwired: 4 in]
        n210 = call "PADMINI_AUTO_CYCLE VALUE 70.vi"("Enum"=enum16{"Read", "Write"}."Write", "error in (no error)"=w670, "Input"=w668) -> ("error out"=w669:errorcluster)  [unwired: 7 in, 1 out]
        n211 = call-poly <vilib>:"read DB.vi"("Item offset [byte]"=u32 16, "String length reserved in DB (default=254)"=u16 50, "error in (no error)"=w669, "items #"=u16 1 ("Items # [byte]"), "Data Block #"=w622, "S7 Connection in"=w676) -> ("error out"=w627:errorcluster, "STRING result Array"=w626:string[], "S7 Connection out"=w628:T4)  [unwired: 2 in, 1 out]
        n212 = call-poly <vilib>:"read DB.vi"("Item offset [byte]"=u32 68, "String length reserved in DB (default=254)"=u16 10, "error in (no error)"=w627, "items #"=u16 1 ("Items # [byte]"), "Data Block #"=w622, "S7 Connection in"=w628) -> ("error out"=w629:errorcluster, "STRING result Array"=w630:string[], "S7 Connection out"=w623:T4)  [unwired: 2 in, 1 out]
        n213 = Build Array (concatenate)(w626, w630) -> (w624:string[])
        n214 = call "PADMINI_AUTO_BARCODE_STRING 70.vi"("Enum"=enum16{"Read", "Write"}."Write", "error in (no error)"=w629, "Input"=w624) -> ("error out"=w649:errorcluster)  [unwired: 7 in, 1 out]
        n215 = global read "DATA LOG.vi" "OP 80 Outputs"() -> (w650:bool)
        n216 = case shown="True" w650 {
          tunnel: [w708 w711] -> w621
          tunnel: [w707 w712] -> w597
          tunnel: w649 -> [w708 w718]
          tunnel: w623 -> [w707 w715]
          frame False {
          }
          frame True {
            w721 = u16 83  # Data Block #
            n217 = call "PADMINI_AUTO_BARCODE_STATUS 80.vi"("Enum"=enum16{"Read", "Write"}."Read", "error in (no error)"=w718) -> ("error out"=w717:errorcluster, "O/P"=w719:i32[])  [unwired: 8 in]
            n218 = global write "DATA LOG.vi" "OP 80 Outputs"(FALSE) -> ()
            n219 = call-poly <vilib>:"write DB.vi"("DINT input array"=w719, "error in (no error)"=w717, "Data Block #"=w721, "S7 Connection in"=w715) -> ("error out"=w709:errorcluster, "S7 Connection out"=w710:T4)  [unwired: 4 in, 2 out]
            n220 = call-poly <vilib>:"write DB.vi"("DINT input array"=i32[] [0] ("Data Byte"), "error in (no error)"=w709, "Data Block #"=u16 82, "S7 Connection in"=w710) -> ("error out"=w711:errorcluster, "S7 Connection out"=w712:T4)  [unwired: 4 in, 2 out]
          }
        }
        n221 = global read "DATA LOG.vi" "OP 80 reset"() -> (w620:bool)
        n222 = global read "DATA LOG.vi" "Auto Cycle On"() -> (w595:bool)
        n223 = case shown="True" w620 {
          tunnel: w621 -> [w688 w696]
          tunnel: [w688 w691] -> _
          tunnel: [w688 w691] -> w610
          tunnel: w597 -> [w687 w690]
          tunnel: [w687 w689] -> w596
          frame False {
          }
          frame True {
            n224 = global write "DATA LOG.vi" "OP 80 reset"(FALSE) -> ()
            n225 = call-poly <vilib>:"write DB.vi"("Item offset [byte]"=u16 4 ("Data Block #"), "DINT input array"=i32[] [0], "error in (no error)"=w696, "Data Block #"=u16 82, "S7 Connection in"=w690) -> ("error out"=w691:errorcluster, "S7 Connection out"=w689:T4)  [unwired: 3 in, 2 out]
          }
        }
        n226 = Boolean To (0,1)(Boolean=w595) -> (0, 1=w594:i16)
        n227 = Build Array(w594) -> (w593:i16[])
        n228 = global read "Global 1.vi" "Filtered BARCODE selected"() -> (w613:string[])
        n229 = call-poly <vilib>:"write DB.vi"("Item offset [byte]"=u32 20, "DINT input array"=w593, "error in (no error)"=w610, "Data Block #"=w616, "S7 Connection in"=w596) -> ("error out"=w618:errorcluster, "S7 Connection out"=w619:T4)  [unwired: 3 in, 2 out]
        n230 = call-poly <vilib>:"write DB.vi"("Item offset [byte]"=u32 24, "Input STRINGS"=w613, "error in (no error)"=w618, "String length reserved in DB (default=254)"=u16 15, "Data Block #"=w616, "S7 Connection in"=w619) -> ("error out"=w611:errorcluster, "S7 Connection out"=w612:T4)  [unwired: 2 in, 2 out]
        n231 = call-poly <vilib>:"read DB.vi"("error in (no error)"=w611, "items #"=u16 2 ("Items # [byte]"), "Data Block #"=w599, "S7 Connection in"=w612) -> ("error out"=w652:errorcluster, "DINT result array"=w654:i32[], "S7 Connection out"=w657:T4)  [unwired: 5 in]
        n232 = call "PADMINI_AUTO_CYCLE STATE 80.vi"("Enum"=enum16{"Read", "Write"}."Write", "error in (no error)"=w652, "Input"=w654) -> ("error out"=w656:errorcluster)  [unwired: 7 in, 1 out]
        n233 = call-poly <vilib>:"read DB.vi"("Item offset [byte]"=u32 8, "error in (no error)"=w656, "items #"=u16 1 ("Items # [byte]"), "Data Block #"=w599, "S7 Connection in"=w657) -> ("error out"=w664:errorcluster, "REAL result array"=w666:sgl[], "S7 Connection out"=w658:T4)  [unwired: 4 in]
        n234 = call "PADMINI_AUTO_CYCLE VALUE 80.vi"("Enum"=enum16{"Read", "Write"}."Write", "error in (no error)"=w664, "Input"=w666) -> ("error out"=w665:errorcluster)  [unwired: 7 in, 1 out]
        n235 = call-poly <vilib>:"read DB.vi"("Item offset [byte]"=u32 12, "String length reserved in DB (default=254)"=u16 50, "error in (no error)"=w665, "items #"=u16 1 ("Items # [byte]"), "Data Block #"=w599, "S7 Connection in"=w658) -> ("error out"=w605:errorcluster, "STRING result Array"=w603:string[], "S7 Connection out"=w601:T4)  [unwired: 2 in, 1 out]
        n236 = call-poly <vilib>:"read DB.vi"("Item offset [byte]"=u32 64, "String length reserved in DB (default=254)"=u16 10, "error in (no error)"=w605, "items #"=u16 2 ("Items # [byte]"), "Data Block #"=w599, "S7 Connection in"=w601) -> ("error out"=w604:errorcluster, "STRING result Array"=w609:string[], "S7 Connection out"=w600:T4)  [unwired: 2 in, 1 out]
        n237 = Build Array (concatenate)(w603, w609) -> (w602:string[])
        n238 = call "PADMINI_AUTO_BARCODE_STRING 80.vi"("Enum"=enum16{"Read", "Write"}."Write", "error in (no error)"=w604, "Input"=w602) -> ("error out"=w648:errorcluster)  [unwired: 7 in, 1 out]
      }
      frame #1 {
        # "RECONNECT"
        n239 = case shown="Error" w740 {
          selector: w740 -> [w745 w753]
          tunnel: [w744 w750] -> w738
          tunnel: [w745 w751] -> w739
          tunnel: w741 -> [w744 w747]
          tunnel: w737 -> [_ w746]
          frame No Error {
          }
          frame Error {
            n240 = call <vilib>:"Clear Errors.vi"("error in (no error)"=w753) -> ("error out"=w754:errorcluster)  [unwired: 5 in, 1 out]
            n241 = call <vilib>:"disconnect.vi"("error in (no error)"=w754, "S7 Connection in"=w747) -> ("error out"=w752:errorcluster)  [unwired: 8 in, 1 out]
            n242 = call <vilib>:"Clear Errors.vi"("error in (no error)"=w752) -> ("error out"=w749:errorcluster)  [unwired: 5 in, 1 out]
            n243 = call <vilib>:"connect.vi"("PLC Type"=PLC_Type."S7 1200" ("PLC Type 2"), "error in (no error)"=w749, "IP address"=w746) -> ("error out"=w751:errorcluster, "S7 Connection out"=w750:T4)  [unwired: 7 in]
          }
        }
        n244 = Unbundle By Name(w740) -> ("status"=w743:bool)
        n245 = Not(x=w743) -> (.not. x?=w742:bool)
        "PLC 6" <- w742
        n246 = global write "Global 1.vi" "PLC 6"(w742) -> ()
      }
    }
    n247 = call "PADMINI_STOP_ALL.vi"("Enum"=enum16{"Read", "Write"}."Read") -> ("Boolean 2"=w583:bool)  [unwired: 9 in, 1 out]
    n248 = local read "stop"() -> (w582:bool)
    n249 = Or(x=w582, y=w583) -> (x .or. y?=w581:bool)
    n250 = Wait (ms)(milliseconds to wait=u32 50) -> ()  [unwired: 1 out]
  }
  n251 = while {
    shift-right: [w757] -> w72
    shift-left: w75 -> [w767]
    shift-right: [w765] -> w73
    shift-left: w76 -> [w766]
    tunnel: w71 -> [w756]
    stop <- w759 stop-if-true
    # "OP 60"
    n252 = flat-sequence {
      tunnel: [w776] -> w763
      tunnel: [w798] -> w758
      tunnel: w766 -> [w817]
      tunnel: w767 -> [w816]
      tunnel: w756 -> [w797]
      tunnel: [w797] -> w755
      tunnel: [w845] -> w765
      tunnel: [w844] -> w757
      tunnel: w763 -> [w847]
      tunnel: w758 -> [w846]
      tunnel: w755 -> [w843]
      frame #0 {
        w793 = u16 44 ("Data Block #")
        w773 = u16 43 ("Data Block #")
        # "AUTO WRITE"
        n253 = global read "DATA LOG.vi" "OP 60 Outputs"() -> (w815:bool)
        n254 = case shown="True" w815 {
          tunnel: w816 -> [w828 w841]
          tunnel: [w829 w830] -> w785
          tunnel: [w828 w833] -> w784
          tunnel: w817 -> [w829 w838]
          frame False {
          }
          frame True {
            w842 = u16 44  # Data Block #
            n255 = call "PADMINI_AUTO_BARCODE_STATUS 60.vi"("Enum"=enum16{"Read", "Write"}."Read", "error in (no error)"=w838) -> ("error out"=w837:errorcluster, "O/P"=w839:i32[])  [unwired: 8 in]
            n256 = global write "DATA LOG.vi" "OP 60 Outputs"(FALSE) -> ()
            n257 = call-poly <vilib>:"write DB.vi"("DINT input array"=w839, "error in (no error)"=w837, "Data Block #"=w842, "S7 Connection in"=w841) -> ("error out"=w831:errorcluster, "S7 Connection out"=w832:T4)  [unwired: 4 in, 2 out]
            n258 = call-poly <vilib>:"write DB.vi"("DINT input array"=i32[] [0] ("Data Byte"), "error in (no error)"=w831, "Data Block #"=u16 43, "S7 Connection in"=w832) -> ("error out"=w830:errorcluster, "S7 Connection out"=w833:T4)  [unwired: 4 in, 2 out]
          }
        }
        n259 = global read "DATA LOG.vi" "OP 60 reset"() -> (w783:bool)
        n260 = global read "DATA LOG.vi" "Auto Cycle On"() -> (w770:bool)
        n261 = case shown="True" w783 {
          tunnel: w785 -> [w818 w827]
          tunnel: [w818 w826] -> w786
          tunnel: w784 -> [w819 w825]
          tunnel: [w819 w824] -> w787
          frame False {
          }
          frame True {
            n262 = global write "DATA LOG.vi" "OP 60 reset"(FALSE) -> ()
            n263 = call-poly <vilib>:"write DB.vi"("Item offset [byte]"=u16 4 ("Data Block #"), "DINT input array"=i32[] [0], "error in (no error)"=w827, "Data Block #"=u16 43, "S7 Connection in"=w825) -> ("error out"=w826:errorcluster, "S7 Connection out"=w824:T4)  [unwired: 3 in, 2 out]
          }
        }
        n264 = Boolean To (0,1)(Boolean=w770) -> (0, 1=w769:i16)
        n265 = Build Array(w769) -> (w768:i16[])
        n266 = global read "Global 1.vi" "Filtered BARCODE selected"() -> (w796:string[])
        n267 = call-poly <vilib>:"write DB.vi"("Item offset [byte]"=u32 20, "DINT input array"=w768, "error in (no error)"=w786, "Data Block #"=w793, "S7 Connection in"=w787) -> ("error out"=w791:errorcluster, "S7 Connection out"=w790:T4)  [unwired: 3 in, 2 out]
        n268 = call-poly <vilib>:"write DB.vi"("Item offset [byte]"=u32 24, "Input STRINGS"=w796, "error in (no error)"=w791, "String length reserved in DB (default=254)"=u16 15, "Data Block #"=w793, "S7 Connection in"=w790) -> ("error out"=w788:errorcluster, "S7 Connection out"=w789:T4)  [unwired: 2 in, 2 out]
        n269 = call-poly <vilib>:"read DB.vi"("error in (no error)"=w788, "items #"=u16 2 ("Items # [byte]"), "Data Block #"=w773, "S7 Connection in"=w789) -> ("error out"=w813:errorcluster, "DINT result array"=w811:i32[], "S7 Connection out"=w808:T4)  [unwired: 5 in]
        n270 = call "PADMINI_AUTO_CYCLE STATE 60.vi"("Enum"=enum16{"Read", "Write"}."Write", "error in (no error)"=w813, "Input"=w811) -> ("error out"=w809:errorcluster)  [unwired: 7 in, 1 out]
        n271 = call-poly <vilib>:"read DB.vi"("Item offset [byte]"=u32 8, "error in (no error)"=w809, "items #"=u16 6 ("Items # [byte]"), "Data Block #"=w773, "S7 Connection in"=w808) -> ("error out"=w801:errorcluster, "REAL result array"=w799:sgl[], "S7 Connection out"=w807:T4)  [unwired: 4 in]
        n272 = call "PADMINI_AUTO_CYCLE VALUE 60.vi"("Enum"=enum16{"Read", "Write"}."Write", "error in (no error)"=w801, "Input"=w799) -> ("error out"=w800:errorcluster)  [unwired: 7 in, 1 out]
        n273 = call-poly <vilib>:"read DB.vi"("Item offset [byte]"=u32 32, "String length reserved in DB (default=254)"=u16 50, "error in (no error)"=w800, "items #"=u16 1 ("Items # [byte]"), "Data Block #"=w773, "S7 Connection in"=w807) -> ("error out"=w778:errorcluster, "STRING result Array"=w775:string[], "S7 Connection out"=w777:T4)  [unwired: 2 in, 1 out]
        n274 = call-poly <vilib>:"read DB.vi"("Item offset [byte]"=u32 84, "String length reserved in DB (default=254)"=u16 10, "error in (no error)"=w778, "items #"=u16 7 ("Items # [byte]"), "Data Block #"=w773, "S7 Connection in"=w777) -> ("error out"=w779:errorcluster, "STRING result Array"=w782:string[], "S7 Connection out"=w776:T4)  [unwired: 2 in, 1 out]
        n275 = Build Array (concatenate)(w775, w782) -> (w774:string[])
        n276 = call "PADMINI_AUTO_BARCODE_STRING 60.vi"("Enum"=enum16{"Read", "Write"}."Write", "error in (no error)"=w779, "Input"=w774) -> ("error out"=w798:errorcluster)  [unwired: 7 in, 1 out]
      }
      frame #1 {
        # "RECONNECT"
        n277 = case shown="Error" w846 {
          selector: w846 -> [w851 w859]
          tunnel: [w850 w856] -> w844
          tunnel: [w851 w857] -> w845
          tunnel: w847 -> [w850 w853]
          tunnel: w843 -> [_ w852]
          frame No Error {
          }
          frame Error {
            n278 = call <vilib>:"Clear Errors.vi"("error in (no error)"=w859) -> ("error out"=w860:errorcluster)  [unwired: 5 in, 1 out]
            n279 = call <vilib>:"disconnect.vi"("error in (no error)"=w860, "S7 Connection in"=w853) -> ("error out"=w858:errorcluster)  [unwired: 8 in, 1 out]
            n280 = call <vilib>:"Clear Errors.vi"("error in (no error)"=w858) -> ("error out"=w855:errorcluster)  [unwired: 5 in, 1 out]
            n281 = call <vilib>:"connect.vi"("PLC Type"=PLC_Type."S7 1200" ("PLC Type 2"), "error in (no error)"=w855, "IP address"=w852) -> ("error out"=w857:errorcluster, "S7 Connection out"=w856:T4)  [unwired: 7 in]
          }
        }
        n282 = Unbundle By Name(w846) -> ("status"=w849:bool)
        n283 = Not(x=w849) -> (.not. x?=w848:bool)
        "PLC 5" <- w848
        n284 = global write "Global 1.vi" "PLC 5"(w848) -> ()
      }
    }
    n285 = call "PADMINI_STOP_ALL.vi"("Enum"=enum16{"Read", "Write"}."Read") -> ("Boolean 2"=w761:bool)  [unwired: 9 in, 1 out]
    n286 = local read "stop"() -> (w760:bool)
    n287 = Or(x=w760, y=w761) -> (x .or. y?=w759:bool)
    n288 = Wait (ms)(milliseconds to wait=u32 50) -> ()  [unwired: 1 out]
  }
  n289 = while {
    shift-right: [w863] -> w110
    shift-left: w114 -> [w873]
    shift-right: [w871] -> w111
    shift-left: w115 -> [w872]
    tunnel: w113 -> [w862]
    stop <- w865 stop-if-true
    # "OP 40"
    n290 = flat-sequence {
      tunnel: [w885] -> w869
      tunnel: [w904] -> w864
      tunnel: w872 -> [w923]
      tunnel: w873 -> [w922]
      tunnel: w862 -> [w903]
      tunnel: [w903] -> w861
      tunnel: [w951] -> w871
      tunnel: [w950] -> w863
      tunnel: w869 -> [w953]
      tunnel: w864 -> [w952]
      tunnel: w861 -> [w949]
      frame #0 {
        w896 = u16 57 ("Data Block #")
        w884 = u16 56 ("Data Block #")
        # "AUTO WRITE"
        n291 = global read "DATA LOG.vi" "OP 40 Outputs"() -> (w921:bool)
        n292 = case shown="True" w921 {
          tunnel: w922 -> [w934 w947]
          tunnel: [w935 w939] -> w901
          tunnel: [w934 w941] -> w902
          tunnel: w923 -> [w935 w944]
          frame False {
          }
          frame True {
            w948 = u16 57  # Data Block #
            n293 = call "PADMINI_AUTO_BARCODE_STATUS 40.vi"("Enum"=enum16{"Read", "Write"}."Read", "error in (no error)"=w944) -> ("error out"=w943:errorcluster, "O/P"=w945:i32[])  [unwired: 8 in]
            n294 = global write "DATA LOG.vi" "OP 40 Outputs"(FALSE) -> ()
            n295 = call-poly <vilib>:"write DB.vi"("DINT input array"=w945, "error in (no error)"=w943, "Data Block #"=w948, "S7 Connection in"=w947) -> ("error out"=w938:errorcluster, "S7 Connection out"=w940:T4)  [unwired: 4 in, 2 out]
            n296 = call-poly <vilib>:"write DB.vi"("DINT input array"=i32[] [0], "error in (no error)"=w938, "Data Block #"=u16 56, "S7 Connection in"=w940) -> ("error out"=w939:errorcluster, "S7 Connection out"=w941:T4)  [unwired: 4 in, 2 out]
          }
        }
        n297 = global read "DATA LOG.vi" "OP 40 reset"() -> (w900:bool)
        n298 = global read "DATA LOG.vi" "Auto Cycle On"() -> (w876:bool)
        n299 = case shown="True" w900 {
          tunnel: w901 -> [w924 w933]
          tunnel: [w924 w932] -> w889
          tunnel: w902 -> [w925 w931]
          tunnel: [w925 w930] -> w890
          frame False {
          }
          frame True {
            n300 = global write "DATA LOG.vi" "OP 40 reset"(FALSE) -> ()
            n301 = call-poly <vilib>:"write DB.vi"("Item offset [byte]"=u16 4 ("Data Block #"), "DINT input array"=i32[] [0], "error in (no error)"=w933, "Data Block #"=u16 56, "S7 Connection in"=w931) -> ("error out"=w932:errorcluster, "S7 Connection out"=w930:T4)  [unwired: 3 in, 2 out]
          }
        }
        n302 = Boolean To (0,1)(Boolean=w876) -> (0, 1=w875:i16)
        n303 = Build Array(w875) -> (w874:i16[])
        n304 = global read "Global 1.vi" "Filtered BARCODE selected"() -> (w899:string[])
        n305 = call-poly <vilib>:"write DB.vi"("Item offset [byte]"=u32 20, "DINT input array"=w874, "error in (no error)"=w889, "Data Block #"=w896, "S7 Connection in"=w890) -> ("error out"=w894:errorcluster, "S7 Connection out"=w893:T4)  [unwired: 3 in, 2 out]
        n306 = call-poly <vilib>:"write DB.vi"("Item offset [byte]"=u32 24, "Input STRINGS"=w899, "error in (no error)"=w894, "String length reserved in DB (default=254)"=u16 15, "Data Block #"=w896, "S7 Connection in"=w893) -> ("error out"=w891:errorcluster, "S7 Connection out"=w892:T4)  [unwired: 2 in, 2 out]
        n307 = call-poly <vilib>:"read DB.vi"("error in (no error)"=w891, "items #"=u16 2 ("Items # [byte]"), "Data Block #"=w884, "S7 Connection in"=w892) -> ("error out"=w919:errorcluster, "DINT result array"=w917:i32[], "S7 Connection out"=w914:T4)  [unwired: 5 in]
        n308 = call "PADMINI_AUTO_CYCLE STATE 40.vi"("Enum"=enum16{"Read", "Write"}."Write", "error in (no error)"=w919, "Input"=w917) -> ("error out"=w915:errorcluster)  [unwired: 7 in, 1 out]
        n309 = call-poly <vilib>:"read DB.vi"("Item offset [byte]"=u32 8, "error in (no error)"=w915, "items #"=u16 4 ("Items # [byte]"), "Data Block #"=w884, "S7 Connection in"=w914) -> ("error out"=w907:errorcluster, "REAL result array"=w905:sgl[], "S7 Connection out"=w913:T4)  [unwired: 4 in]
        n310 = call "PADMINI_AUTO_CYCLE VALUE 40.vi"("Enum"=enum16{"Read", "Write"}."Write", "error in (no error)"=w907, "Input"=w905) -> ("error out"=w906:errorcluster)  [unwired: 7 in, 1 out]
        n311 = call-poly <vilib>:"read DB.vi"("Item offset [byte]"=u32 24, "String length reserved in DB (default=254)"=u16 50, "error in (no error)"=w906, "items #"=u16 1 ("Items # [byte]"), "Data Block #"=w884, "S7 Connection in"=w913) -> ("error out"=w888:errorcluster, "STRING result Array"=w879:string[], "S7 Connection out"=w886:T4)  [unwired: 2 in, 1 out]
        n312 = call-poly <vilib>:"read DB.vi"("Item offset [byte]"=u32 76, "String length reserved in DB (default=254)"=u16 10, "error in (no error)"=w888, "items #"=u16 4 ("Items # [byte]"), "Data Block #"=w884, "S7 Connection in"=w886) -> ("error out"=w887:errorcluster, "STRING result Array"=w878:string[], "S7 Connection out"=w885:T4)  [unwired: 2 in, 1 out]
        n313 = Build Array (concatenate)(w879, w878) -> (w877:string[])
        n314 = call "PADMINI_AUTO_BARCODE_STRING 40.vi"("Enum"=enum16{"Read", "Write"}."Write", "error in (no error)"=w887, "Input"=w877) -> ("error out"=w904:errorcluster)  [unwired: 7 in, 1 out]
      }
      frame #1 {
        # "RECONNECT"
        n315 = case shown="Error" w952 {
          selector: w952 -> [w957 w965]
          tunnel: [w956 w962] -> w950
          tunnel: [w957 w963] -> w951
          tunnel: w953 -> [w956 w959]
          tunnel: w949 -> [_ w958]
          frame No Error {
          }
          frame Error {
            n316 = call <vilib>:"Clear Errors.vi"("error in (no error)"=w965) -> ("error out"=w966:errorcluster)  [unwired: 5 in, 1 out]
            n317 = call <vilib>:"disconnect.vi"("error in (no error)"=w966, "S7 Connection in"=w959) -> ("error out"=w964:errorcluster)  [unwired: 8 in, 1 out]
            n318 = call <vilib>:"Clear Errors.vi"("error in (no error)"=w964) -> ("error out"=w961:errorcluster)  [unwired: 5 in, 1 out]
            n319 = call <vilib>:"connect.vi"("PLC Type"=PLC_Type."S7 1200" ("PLC Type 2"), "error in (no error)"=w961, "IP address"=w958) -> ("error out"=w963:errorcluster, "S7 Connection out"=w962:T4)  [unwired: 7 in]
          }
        }
        n320 = Unbundle By Name(w952) -> ("status"=w955:bool)
        n321 = Not(x=w955) -> (.not. x?=w954:bool)
        "PLC 3" <- w954
        n322 = global write "Global 1.vi" "PLC 3"(w954) -> ()
      }
    }
    n323 = call "PADMINI_STOP_ALL.vi"("Enum"=enum16{"Read", "Write"}."Read") -> ("Boolean 2"=w867:bool)  [unwired: 9 in, 1 out]
    n324 = local read "stop"() -> (w866:bool)
    n325 = Or(x=w866, y=w867) -> (x .or. y?=w865:bool)
    n326 = Wait (ms)(milliseconds to wait=u32 50) -> ()  [unwired: 1 out]
  }
  n327 = call <vilib>:"Clear Errors.vi"("error in (no error)"=w111) -> ("error out"=w112:errorcluster)  [unwired: 5 in, 1 out]
  n328 = call <vilib>:"Clear Errors.vi"("error in (no error)"=w120) -> ("error out"=w122:errorcluster)  [unwired: 5 in, 1 out]
  n329 = call <vilib>:"Clear Errors.vi"("error in (no error)"=w95) -> ("error out"=w94:errorcluster)  [unwired: 5 in, 1 out]
  n330 = call <vilib>:"Clear Errors.vi"("error in (no error)"=w73) -> ("error out"=w74:errorcluster)  [unwired: 5 in, 1 out]
  n331 = call <vilib>:"disconnect.vi"("error in (no error)"=w112, "S7 Connection in"=w110) -> ("error out"=w109:errorcluster)  [unwired: 8 in, 1 out]
  n332 = call <vilib>:"disconnect.vi"("error in (no error)"=w122, "S7 Connection in"=w121) -> ("error out"=w108:errorcluster)  [unwired: 8 in, 1 out]
  n333 = call <vilib>:"disconnect.vi"("error in (no error)"=w94, "S7 Connection in"=w96) -> ("error out"=w70:errorcluster)  [unwired: 8 in, 1 out]
  n334 = call <vilib>:"disconnect.vi"("error in (no error)"=w74, "S7 Connection in"=w72) -> ("error out"=w69:errorcluster)  [unwired: 8 in, 1 out]
  n335 = Merge Errors(w108, w109, w70, w69) -> (w107:errorcluster)
  n336 = call <vilib>:"Clear Errors.vi"("error in (no error)"=w53) -> ("error out"=w54:errorcluster)  [unwired: 5 in, 1 out]
  n337 = call <vilib>:"disconnect.vi"("error in (no error)"=w54, "S7 Connection in"=w52) -> ("error out"=w22:errorcluster)  [unwired: 8 in, 1 out]
  n338 = call <vilib>:"Clear Errors.vi"("error in (no error)"=w163) -> ("error out"=w149:errorcluster)  [unwired: 5 in, 1 out]
  n339 = call <vilib>:"disconnect.vi"("error in (no error)"=w149, "S7 Connection in"=w148) -> ("error out"=w147:errorcluster)  [unwired: 8 in, 1 out]
  n340 = control-ref of="This VI"() -> (w3:refnum<vi>)
  n341 = call <vilib>:"Clear Errors.vi"("error in (no error)"=w24) -> ("error out"=w25:errorcluster)  [unwired: 5 in, 1 out]
  n342 = call <vilib>:"disconnect.vi"("error in (no error)"=w25, "S7 Connection in"=w23) -> ("error out"=w20:errorcluster)  [unwired: 8 in, 1 out]
  n343 = Merge Errors(w22, w20) -> (w21:errorcluster)
  n344 = Merge Errors(w147, w107, w21) -> (w168:errorcluster)
  n345 = call <vilib>:"Simple Error Handler.vi"("type of dialog (OK msg:1)"=w2, "error in (no error)"=w168) -> ("error out"=w167:errorcluster)  [unwired: 3 in, 4 out]
  n346 = call <vilib>:"Clear Errors.vi"("error in (no error)"=w167) -> ("error out"=w166:errorcluster)  [unwired: 5 in, 1 out]
  n347 = invoke class="VI" method="FP.Close"(reference=w3, error in=w166) -> (error out=→"error out":errorcluster)  [unwired: 1 in, 2 out]
